vi "Set illumination arm.vi"(8 "error in (no error)":errorcluster, 11 "AOTF in":refnum<class "AOTF.lvclass">) -> (0 "error out":errorcluster, 3 "AOTF out":refnum<class "AOTF.lvclass">)   [LabVIEW 2012, in "AOTF.lvclass"]
uses:
  AOTF.lvclass
  AOTF.lvclass/AOTF.ctl
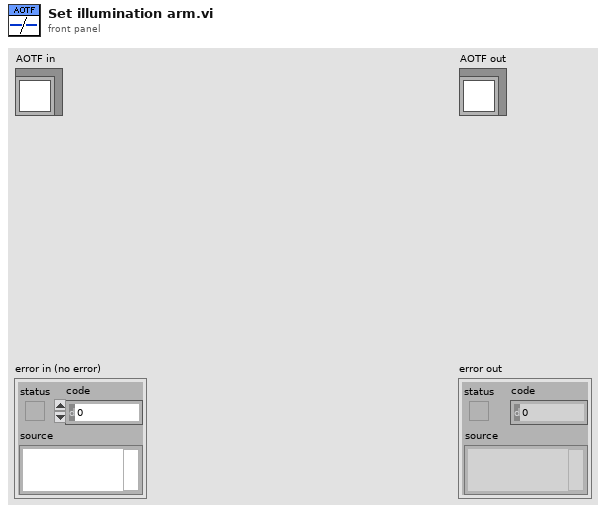
[diagram p1: front panel]
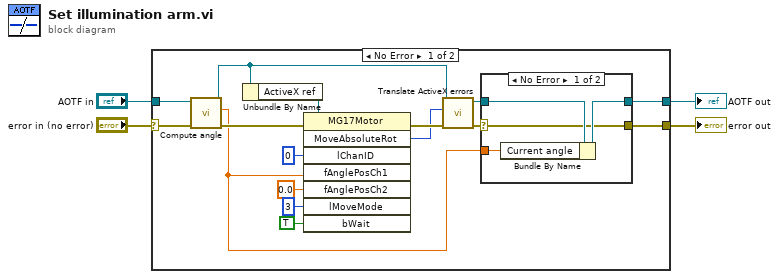
[diagram p0: block diagram]
diagram:
  n1 = case shown="No Error" "error in (no error)" {
    selector: "error in (no error)" -> [w15 w28]
    tunnel: [w5 w28] -> w3
    tunnel: [w9 w27] -> w1
    tunnel: "AOTF in" -> [w16 w27]
    frame No Error {
      n2 = call-dynamic "Compute angle.vi"("error in (no error)"=w15, "AOTF in"=w16) -> ("error out"=w14:errorcluster, "Angle"=w6:sgl, "AOTF out"=w10:refnum<class "AOTF.lvclass">)  [unwired: 7 in]
      n3 = Unbundle By Name(w10) -> ("ActiveX ref"=w20:refnum<k7>)
      n4 = invoke class="MG17Motor" method="MoveAbsoluteRot"(reference=w20, error in=w14, "lChanID"=0, "fAnglePosCh1"=w6, "fAnglePosCh2"=sgl 0.0, "lMoveMode"=3, "bWait"=TRUE) -> (error out=w13:errorcluster, "MoveAbsoluteRot"=w8:i32)  [unwired: 1 in, 6 out]
      n5 = call-dynamic "Translate ActiveX errors.vi"("error in (no error)"=w13, "ActiveX return"=w8, "AOTF in"=w10) -> ("error out"=w7:errorcluster, "AOTF out"=w11:refnum<class "AOTF.lvclass">)  [unwired: 7 in]
      n6 = case shown="No Error" w7 {
        selector: w7 -> [w21 w25]
        tunnel: w11 -> [w24 w26]
        tunnel: [w23 w26] -> w9
        tunnel: w6 -> [w22 _]
        tunnel: [w21 w25] -> w5
        frame No Error {
          n7 = Bundle By Name(cluster=w24, "Current angle"=w22) -> (w23:refnum<class "AOTF.lvclass">)
        }
        frame Error {
        }
      }
    }
    frame Error {
    }
  }
  "error out" <- w3
  "AOTF out" <- w1
